vi "nanocal -- nuclear schottky fit V5.vi"() -> ()   [LabVIEW 2020] (continued)
\"mm3\" -> 0.000000000000   ,  \"T\" -> 1.000000000000   ,  \"B\" -> 0.000000000000   ,  \"θ\" -> 0.000000000000   ,  \"Reoff\" -> 0.000000000000   ,  \"Imoff\" -> 0.000000000000    |>   , \r\"IDS0220_210310_RAW_cal__ref_\" ->   <|    \"ζ\" -> 0.000000000000   ,  \"τ1\" -> 0.000000000000   ,  \"τS\" -> 0.000000000000   ,  \"τN\" -> 0.000000000000   ,  \"τC\" -> 0.000000000000   ,  \"κ0\" -> 0.000000000000   ,  \"mm1\" -> 0.000000000000   ,  \"mm2\" -> 0.000000000000   ,  \"mm3\" -> 0.000000000000   ,  \"T\" -> 0.677000000000   ,  \"B\" -> 0.000000000000   ,  \"θ\" -> 0.000000000000   ,  \"Reoff\" -> 0.000000000000   ,  \"Imoff\" -> 0.000000000000    |>   , \r\"IDS0220_210310_RAW_cal__sam_\" ->   <|    \"ζ\" -> 0.000000000000   ,  \"τ1\" -> 0.000000000000   ,  \"τS\" -> 0.000000000000   ,  \"τN\" -> 0.000000000000   ,  \"τC\" -> 0.000000000000   ,  \"κ0\" -> 0.000000000000   ,  \"mm1\" -> 0.000000000000   ,  \"mm2\" -> 0.000000000000   ,  \"mm3\" -> 0.000000000000   ,  \"T\" -> 0.677000000000   ,  \"B\" -> 0.000000000000   ,  \"θ\" -> 0.000000000000   ,  \"Reoff\" -> 0.000000000000   ,  \"Imoff\" -> 0.000000000000    |>   , \r\"IDS0224_210310_RAW_cal__ref_\" ->   <|    \"ζ\" -> 0.000000000000   ,  \"τ1\" -> 0.000000000000   ,  \"τS\" -> 0.000000000000   ,  \"τN\" -> 0.000000000000   ,  \"τC\" -> 0.000000000000   ,  \"κ0\" -> 0.000000000000   ,  \"mm1\" -> 0.000000000000   ,  \"mm2\" -> 0.000000000000   ,  \"mm3\" -> 0.000000000000   ,  \"T\" -> 0.000000000000   ,  \"B\" -> 0.000000000000   ,  \"θ\" -> 0.000000000000   ,  \"Reoff\" -> 0.000000000000   ,  \"Imoff\" -> 0.000000000000    |>   , \r\"IDS0224_210310_RAW_cal__sam_\" ->   <|    \"ζ\" -> 0.000000000000   ,  \"τ1\" -> 0.000000000000   ,  \"τS\" -> 0.000000000000   ,  \"τN\" -> 0.000000000000   ,  \"τC\" -> 0.000000000000   ,  \"κ0\" -> 0.000000000000   ,  \"mm1\" -> 0.000000000000   ,  \"mm2\" -> 0.000000000000   ,  \"mm3\" -> 0.000000000000   ,  \"T\" -> 0.000000000000   ,  \"B\" -> 0.000000000000   ,  \"θ\" -> 0.000000000000   ,  \"Reoff\" -> 0.000000000000   ,  \"Imoff\" -> 0.000000000000    |>   , \r\"IDS0293_210427_RAW_cal__ref_\" ->   <|    \"ζ\" -> 0.016384838586   ,  \"τ1\" -> 0.013784349529   ,  \"τS\" -> 0.011495286759   ,  \"τN\" -> 0.000117117954   ,  \"τC\" -> 0.004048153799   ,  \"κ0\" -> 0.000000013122   ,  \"mm1\" -> 0.000000000000   ,  \"mm2\" -> 0.000000000000   ,  \"mm3\" -> 0.000000000000   ,  \"T\" -> 1.900000000000   ,  \"B\" -> 12.000000000000   ,  \"θ\" -> 30.000000000000   ,  \"Reoff\" -> 0.000000000000   ,  \"Imoff\" -> 0.000000000000    |>   , \r\"IDS0293_210427_RAW_cal__sam_\" ->   <|    \"ζ\" -> 0.009772435939   ,  \"τ1\" -> 0.020827345370   ,  \"τS\" -> 0.013809334085   ,  \"τN\" -> 0.000168485133   ,  \"τC\" -> 0.005555066716   ,  \"κ0\" -> 0.000000013930   ,  \"mm1\" -> 0.000000000000   ,  \"mm2\" -> 0.000000000000   ,  \"mm3\" -> 0.000000000000   ,  \"T\" -> 1.900000000000   ,  \"B\" -> 12.000000000000   ,  \"θ\" -> 30.000000000000   ,  \"Reoff\" -> 0.000000000000   ,  \"Imoff\" -> 0.000000000000    |>   , \r\"IDS0294_210427_RAW_cal__ref_\" ->   <|    \"ζ\" -> 0.017975147456   ,  \"τ1\" -> 0.015573317032   ,  \"τS\" -> 0.016697357463   ,  \"τN\" -> 0.000401487663   ,  \"τC\" -> 0.004243374884   ,  \"κ0\" -> 0.000000007622   ,  \"mm1\" -> 0.000000000000   ,  \"mm2\" -> 0.000000000000   ,  \"mm3\" -> 0.000000000000   ,  \"T\" -> 1.130000000000   ,  \"B\" -> 12.000000000000   ,  \"θ\" -> 30.000000000000   ,  \"Reoff\" -> 0.000000000000   ,  \"Imoff\" -> 0.000000000000    |>   , \r\"IDS0294_210427_RAW_cal__sam_\" ->   <|    \"ζ\" -> 0.010912011148   ,  \"τ1\" -> 0.020760977312   ,  \"τS\" -> 0.021106239637   ,  \"τN\" -> 0.000452316988   ,  \"τC\" -> 0.005003723454   ,  \"κ0\" -> 0.000000008194   ,  \"mm1\" -> 0.000000000000   ,  \"mm2\" -> 0.000000000000   ,  \"mm3\" -> 0.000000000000   ,  \"T\" -> 1.130000000000   ,  \"B\" -> 12.000000000000   ,  \"θ\" -> 30.000000000000   ,  \"Reoff\" -> 0.000000000000   ,  \"Imoff\" -> 0.000000000000    |>   , \r\"IDS0295_210427_RAW_cal__ref_\" ->   <|    \"ζ\" -> 0.021360373560   ,  \"τ1\" -> 0.017226807214   ,  \"τS\" -> 0.021136224671   ,  \"τN\" -> 0.000857882935   ,  \"τC\" -> 0.004088468956   ,  \"κ0\" -> 0.000000005432   ,  \"mm1\" -> 0.000000000000   ,  \"mm2\" -> 0.000000000000   ,  \"mm3\" -> 0.000000000000   ,  \"T\" -> 0.830000000000   ,  \"B\" -> 12.000000000000   ,  \"θ\" -> 30.000000000000   ,  \"Reoff\" -> 0.000000000000   ,  \"Imoff\" -> 0.000000000000    |>   , \r\"IDS0295_210427_RAW_cal__sam_\" ->   <|    \"ζ\" -> 0.013460153434   ,  \"τ1\" -> 0.020684726260   ,  \"τS\" -> 0.027140346721   ,  \"τN\" -> 0.000960302406   ,  \"τC\" -> 0.004517434882   ,  \"κ0\" -> 0.000000005889   ,  \"mm1\" -> 0.000000000000   ,  \"mm2\" -> 0.000000000000   ,  \"mm3\" -> 0.000000000000   ,  \"T\" -> 0.830000000000   ,  \"B\" -> 12.000000000000   ,  \"θ\" -> 30.000000000000   ,  \"Reoff\" -> 0.000000000000   ,  \"Imoff\" -> 0.000000000000    |>   , \r\"IDS0296_210427_RAW_cal__ref_\" ->   <|    \"ζ\" -> 0.027756025784   ,  \"τ1\" -> 0.019742757718   ,  \"τS\" -> 0.026611973171   ,  \"τN\" -> 0.001398943183   ,  \"τC\" -> 0.003482574473   ,  \"κ0\" -> 0.000000003907   ,  \"mm1\" -> 0.000000000000   ,  \"mm2\" -> 0.000000000000   ,  \"mm3\" -> 0.000000000000   ,  \"T\" -> 0.620000000000   ,  \"B\" -> 12.000000000000   ,  \"θ\" -> 30.000000000000   ,  \"Reoff\" -> 0.000000000000   ,  \"Imoff\" -> 0.000000000000    |>   , \r\"IDS0296_210427_RAW_cal__sam_\" ->   <|    \"ζ\" -> 0.016892016292   ,  \"τ1\" -> 0.020344757415   ,  \"τS\" -> 0.033845756966   ,  \"τN\" -> 0.001946817417   ,  \"τC\" -> 0.004013762913   ,  \"κ0\" -> 0.000000004252   ,  \"mm1\" -> 0.000000000000   ,  \"mm2\" -> 0.000000000000   ,  \"mm3\" -> 0.000000000000   ,  \"T\" -> 0.620000000000   ,  \"B\" -> 12.000000000000   ,  \"θ\" -> 30.000000000000   ,  \"Reoff\" -> 0.000000000000   ,  \"Imoff\" -> 0.000000000000    |>   , \r\"IDS0297_210427_RAW_cal__ref_\" ->   <|    \"ζ\" -> 0.034775017342   ,  \"τ1\" -> 0.018923965005   ,  \"τS\" -> 0.030086686370   ,  \"τN\" -> 0.002286572055   ,  \"τC\" -> 0.002714831651   ,  \"κ0\" -> 0.000000003294   ,  \"mm1\" -> 0.000000000000   ,  \"mm2\" -> 0.000000000000   ,  \"mm3\" -> 0.000000000000   ,  \"T\" -> 0.530000000000   ,  \"B\" -> 12.000000000000   ,  \"θ\" -> 30.000000000000   ,  \"Reoff\" -> 0.000000000000   ,  \"Imoff\" -> 0.000000000000    |>   , \r\"IDS0297_210427_RAW_cal__sam_\" ->   <|    \"ζ\" -> 0.021116250068   ,  \"τ1\" -> 0.020669239851   ,  \"τS\" -> 0.037941648749   ,  \"τN\" -> 0.003221866945   ,  \"τC\" -> 0.003619427775   ,  \"κ0\" -> 0.000000003553   ,  \"mm1\" -> 0.000000000000   ,  \"mm2\" -> 0.000000000000   ,  \"mm3\" -> 0.000000000000   ,  \"T\" -> 0.530000000000   ,  \"B\" -> 12.000000000000   ,  \"θ\" -> 30.000000000000   ,  \"Reoff\" -> 0.000000000000   ,  \"Imoff\" -> 0.000000000000    |>   , \r\"IDS0298_210427_RAW_cal__ref_\" ->   <|    \"ζ\" -> 0.046396907778   ,  \"τ1\" -> 0.018912834926   ,  \"τS\" -> 0.034035556993   ,  \"τN\" -> 0.004466176128   ,  \"τC\" -> 0.002290347128   ,  \"κ0\" -> 0.000000002639   ,  \"mm1\" -> 0.000000000000   ,  \"mm2\" -> 0.000000000000   ,  \"mm3\" -> 0.000000000000   ,  \"T\" -> 0.430000000000   ,  \"B\" -> 12.000000000000   ,  \"θ\" -> 30.000000000000   ,  \"Reoff\" -> 0.000000000000   ,  \"Imoff\" -> 0.000000000000    |>   , \r\"IDS0298_210427_RAW_cal__sam_\" ->   <|    \"ζ\" -> 0.028468689077   ,  \"τ1\" -> 0.020220821810   ,  \"τS\" -> 0.043529484347   ,  \"τN\" -> 0.005653540941   ,  \"τC\" -> 0.003150537442   ,  \"κ0\" -> 0.000000002855   ,  \"mm1\" -> 0.000000000000   ,  \"mm2\" -> 0.000000000000   ,  \"mm3\" -> 0.000000000000   ,  \"T\" -> 0.430000000000   ,  \"B\" -> 12.000000000000   ,  \"θ\" -> 30.000000000000   ,  \"Reoff\" -> 0.000000000000   ,  \"Imoff\" -> 0.000000000000    |>   , \r\"IDS0299_210427_RAW_cal__ref_\" ->   <|    \"ζ\" -> 0.060257387765   ,  \"τ1\" -> 0.020933176342   ,  \"τS\" -> 0.038399909631   ,  \"τN\" -> 0.009014166994   ,  \"τC\" -> 0.001999715217   ,  \"κ0\" -> 0.000000002125   ,  \"mm1\" -> 0.000000000000   ,  \"mm2\" -> 0.000000000000   ,  \"mm3\" -> 0.000000000000   ,  \"T\" -> 0.360000000000   ,  \"B\" -> 12.000000000000   ,  \"θ\" -> 30.000000000000   ,  \"Reoff\" -> 0.000000000000   ,  \"Imoff\" -> 0.000000000000    |>   , \r\"IDS0299_210427_RAW_cal__sam_\" ->   <|    \"ζ\" -> 0.036420486357   ,  \"τ1\" -> 0.020986681106   ,  \"τS\" -> 0.049149577509   ,  \"τN\" -> 0.011109585503   ,  \"τC\" -> 0.002819780093   ,  \"κ0\" -> 0.000000002299   ,  \"mm1\" -> 0.000000000000   ,  \"mm2\" -> 0.000000000000   ,  \"mm3\" -> 0.000000000000   ,  \"T\" -> 0.360000000000   ,  \"B\" -> 12.000000000000   ,  \"θ\" -> 30.000000000000   ,  \"Reoff\" -> 0.000000000000   ,  \"Imoff\" -> 0.000000000000    |>   , \r\"IDS0300_210427_RAW_cal__ref_\" ->   <|    \"ζ\" -> 0.338385515343   ,  \"τ1\" -> 0.049005471612   ,  \"τS\" -> 0.154718584573   ,  \"τN\" -> 0.405362096342   ,  \"τC\" -> 0.001218418583   ,  \"κ0\" -> 0.000000000425   ,  \"mm1\" -> 0.000000000000   ,  \"mm2\" -> 0.000000000000   ,  \"mm3\" -> 0.000000000000   ,  \"T\" -> 0.140000000000   ,  \"B\" -> 12.000000000000   ,  \"θ\" -> 30.000000000000   ,  \"Reoff\" -> 0.000000000000   ,  \"Imoff\" -> 0.000000000000    |>   , \r\"IDS0300_210427_RAW_cal__sam_\" ->   <|    \"ζ\" -> 0.211545693132   ,  \"τ1\" -> 0.029106147473   ,  \"τS\" -> 0.094475691604   ,  \"τN\" -> 0.369151052631   ,  \"τC\" -> 0.001396700790   ,  \"κ0\" -> 0.000000000537   ,  \"mm1\" -> 0.000000000000   ,  \"mm2\" -> 0.000000000000   ,  \"mm3\" -> 0.000000000000   ,  \"T\" -> 0.140000000000   ,  \"B\" -> 12.000000000000   ,  \"θ\" -> 30.000000000000   ,  \"Reoff\" -> 0.000000000000   ,  \"Imoff\" -> 0.000000000000    |>   , \r\"IDS0301_210831_RAW_cal__ref_\" ->   <|    \"ζ\" -> 0.083856390991   ,  \"τ1\" -> 0.023882632275   ,  \"τS\" -> 0.042264558819   ,  \"τN\" -> 0.014926022610   ,  \"τC\" -> 0.001493479414   ,  \"κ0\" -> 0.000000001739   ,  \"mm1\" -> 0.000000000000   ,  \"mm2\" -> 0.000000000000   ,  \"mm3\" -> 0.000000000000   ,  \"T\" -> 0.300000000000   ,  \"B\" -> 12.000000000000   ,  \"θ\" -> 30.000000000000   ,  \"Reoff\" -> 0.000000000000   ,  \"Imoff\" -> 0.000000000000    |>   , \r\"IDS0301_210831_RAW_cal__sam_\" ->   <|    \"ζ\" -> 0.050663808076   ,  \"τ1\" -> 0.024940898568   ,  \"τS\" -> 0.056803871413   ,  \"τN\" -> 0.018856862265   ,  \"τC\" -> 0.002133501904   ,  \"κ0\" -> 0.000000001888   ,  \"mm1\" -> 0.000000000000   ,  \"mm2\" -> 0.000000000000   ,  \"mm3\" -> 0.000000000000   ,  \"T\" -> 0.300000000000   ,  \"B\" -> 12.000000000000   ,  \"θ\" -> 30.000000000000   ,  \"Reoff\" -> 0.000000000000   ,  \"Imoff\" -> 0.000000000000    |>   , \r\"IDS0302_210831_RAW_cal__ref_\" ->   <|    \"ζ\" -> 0.118191658932   ,  \"τ1\" -> 0.027786613255   ,  \"τS\" -> 0.049841575379   ,  \"τN\" -> 0.030683320319   ,  \"τC\" -> 0.001300754197   ,  \"κ0\" -> 0.000000001363   ,  \"mm1\" -> 0.000000000000   ,  \"mm2\" -> 0.000000000000   ,  \"mm3\" -> 0.000000000000   ,  \"T\" -> 0.250000000000   ,  \"B\" -> 12.000000000000   ,  \"θ\" -> 30.000000000000   ,  \"Reoff\" -> 0.000000000000   ,  \"Imoff\" -> 0.000000000000    |>   , \r\"IDS0302_210831_RAW_cal__sam_\" ->   <|    \"ζ\" -> 0.072634365939   ,  \"τ1\" -> 0.028637109000   ,  \"τS\" -> 0.065061142288   ,  \"τN\" -> 0.040304243071   ,  \"τC\" -> 0.001622979999   ,  \"κ0\" -> 0.000000001498   ,  \"mm1\" -> 0.000000000000   ,  \"mm2\" -> 0.000000000000   ,  \"mm3\" -> 0.000000000000   ,  \"T\" -> 0.250000000000   ,  \"B\" -> 12.000000000000   ,  \"θ\" -> 30.000000000000   ,  \"Reoff\" -> 0.000000000000   ,  \"Imoff\" -> 0.000000000000    |>   , \r\"IDS0303_210831_RAW_cal__ref_\" ->   <|    \"ζ\" -> 0.210185455037   ,  \"τ1\" -> 0.035884437188   ,  \"τS\" -> 0.076269858590   ,  \"τN\" -> 0.100000000000   ,  \"τC\" -> 0.001092094788   ,  \"κ0\" -> 0.000000001049   ,  \"mm1\" -> 0.000000000000   ,  \"mm2\" -> 0.000000000000   ,  \"mm3\" -> 0.000000000000   ,  \"T\" -> 0.200000000000   ,  \"B\" -> 12.000000000000   ,  \"θ\" -> 30.000000000000   ,  \"Reoff\" -> 0.000000000000   ,  \"Imoff\" -> 0.000000000000    |>   , \r\"IDS0303_210831_RAW_cal__sam_\" ->   <|    \"ζ\" -> 0.128615765969   ,  \"τ1\" -> 0.032665502211   ,  \"τS\" -> 0.082694869013   ,  \"τN\" -> 0.105788373632   ,  \"τC\" -> 0.001439686784   ,  \"κ0\" -> 0.000000001168   ,  \"mm1\" -> 0.000000000000   ,  \"mm2\" -> 0.000000000000   ,  \"mm3\" -> 0.000000000000   ,  \"T\" -> 0.200000000000   ,  \"B\" -> 12.000000000000   ,  \"θ\" -> 30.000000000000   ,  \"Reoff\" -> 0.000000000000   ,  \"Imoff\" -> 0.000000000000    |>   , \r\"IDS0304_210831_RAW_cal__ref_\" ->   <|    \"ζ\" -> 0.270205686716   ,  \"τ1\" -> 0.041964859676   ,  \"τS\" -> 0.093295997771   ,  \"τN\" -> 0.171907220186   ,  \"τC\" -> 0.001079705974   ,  \"κ0\" -> 0.000000000759   ,  \"mm1\" -> 0.000000000000   ,  \"mm2\" -> 0.000000000000   ,  \"mm3\" -> 0.000000000000   ,  \"T\" -> 0.170000000000   ,  \"B\" -> 12.000000000000   ,  \"θ\" -> 30.000000000000   ,  \"Reoff\" -> 0.000000000000   ,  \"Imoff\" -> 0.000000000000    |>   , \r\"IDS0304_210831_RAW_cal__sam_\" ->   <|    \"ζ\" -> 0.156472219566   ,  \"τ1\" -> 0.031017925061   ,  \"τS\" -> 0.080872234530   ,  \"τN\" -> 0.219381306397   ,  \"τC\" -> 0.001437792153   ,  \"κ0\" -> 0.000000000867   ,  \"mm1\" -> 0.000000000000   ,  \"mm2\" -> 0.000000000000   ,  \"mm3\" -> 0.000000000000   ,  \"T\" -> 0.170000000000   ,  \"B\" -> 12.000000000000   ,  \"θ\" -> 30.000000000000   ,  \"Reoff\" -> 0.000000000000   ,  \"Imoff\" -> 0.000000000000    |>   , \r\"IDS0305_210831_RAW_cal__ref_\" ->   <|    \"ζ\" -> 0.288872243536   ,  \"τ1\" -> 0.043051365220   ,  \"τS\" -> 0.113757726379   ,  \"τN\" -> 0.232280670982   ,  \"τC\" -> 0.001075362358   ,  \"κ0\" -> 0.000000000648   ,  \"mm1\" -> 0.000000000000   ,  \"mm2\" -> 0.000000000000   ,  \"mm3\" -> 0.000000000000   ,  \"T\" -> 0.160000000000   ,  \"B\" -> 12.000000000000   ,  \"θ\" -> 30.000000000000   ,  \"Reoff\" -> 0.000000000000   ,  \"Imoff\" -> 0.000000000000    |>   , \r\"IDS0305_210831_RAW_cal__sam_\" ->   <|    \"ζ\" -> 0.162585495535   ,  \"τ1\" -> 0.037883389730   ,  \"τS\" -> 0.086562863191   ,  \"τN\" -> 0.241872534356   ,  \"τC\" -> 0.001506143871   ,  \"κ0\" -> 0.000000000791   ,  \"mm1\" -> 0.000000000000   ,  \"mm2\" -> 0.000000000000   ,  \"mm3\" -> 0.000000000000   ,  \"T\" -> 0.160000000000   ,  \"B\" -> 12.000000000000   ,  \"θ\" -> 30.000000000000   ,  \"Reoff\" -> 0.000000000000   ,  \"Imoff\" -> 0.000000000000    |>   , \r\"IDS0306_210831_RAW_cal__ref_\" ->   <|    \"ζ\" -> 0.013593052641   ,  \"τ1\" -> 0.010989385662   ,  \"τS\" -> 0.007947176041   ,  \"τN\" -> 0.000037757079   ,  \"τC\" -> 0.003572854733   ,  \"κ0\" -> 0.000000023548   ,  \"mm1\" -> 0.000000000000   ,  \"mm2\" -> 0.000000000000   ,  \"mm3\" -> 0.000000000000   ,  \"T\" -> 3.100000000000   ,  \"B\" -> 12.000000000000   ,  \"θ\" -> 30.000000000000   ,  \"Reoff\" -> 0.000000000000   ,  \"Imoff\" -> 0.000000000000    |>   , \r\"IDS0306_210831_RAW_cal__sam_\" ->   <|    \"ζ\" -> 0.010111127240   ,  \"τ1\" -> 0.020788755574   ,  \"τS\" -> 0.009968978424   ,  \"τN\" -> 0.000077788811   ,  \"τC\" -> 0.004598584548   ,  \"κ0\" -> 0.000000024346   ,  \"mm1\" -> 0.000000000000   ,  \"mm2\" -> 0.000000000000   ,  \"mm3\" -> 0.000000000000   ,  \"T\" -> 3.100000000000   ,  \"B\" -> 12.000000000000   ,  \"θ\" -> 30.000000000000   ,  \"Reoff\" -> 0.000000000000   ,  \"Imoff\" -> 0.000000000000    |>   , \r\"IDS0310_210901_RAW_cal__ref_\" ->   <|    \"ζ\" -> 0.308289315544   ,  \"τ1\" -> 0.054346075620   ,  \"τS\" -> 0.066318547481   ,  \"τN\" -> 0.209207967486   ,  \"τC\" -> 0.001005266633   ,  \"κ0\" -> 0.000000000648   ,  \"mm1\" -> 0.000000000000   ,  \"mm2\" -> 0.000000000000   ,  \"mm3\" -> 0.000000000000   ,  \"T\" -> 0.157000000000   ,  \"B\" -> 12.000000000000   ,  \"θ\" -> 45.000000000000   ,  \"Reoff\" -> 0.000000000000   ,  \"Imoff\" -> 0.000000000000    |>   , \r\"IDS0310_210901_RAW_cal__sam_\" ->   <|    \"ζ\" -> 0.295520923520   ,  \"τ1\" -> 0.054772440405   ,  \"τS\" -> 0.071814005451   ,  \"τN\" -> 0.249593767169   ,  \"τC\" -> 0.001103632155   ,  \"κ0\" -> 0.000000000625   ,  \"mm1\" -> 0.000000000000   ,  \"mm2\" -> 0.000000000000   ,  \"mm3\" -> 0.000000000000   ,  \"T\" -> 0.157000000000   ,  \"B\" -> 12.000000000000   ,  \"θ\" -> 45.000000000000   ,  \"Reoff\" -> 0.000000000000   ,  \"Imoff\" -> 0.000000000000    |>   , \r\"IDS0311_210901_RAW_cal__ref_\" ->   <|    \"ζ\" -> 0.509291398058   ,  \"τ1\" -> 0.072489311123   ,  \"τS\" -> 0.090971238975   ,  \"τN\" -> 0.493344947632   ,  \"τC\" -> 0.000983845591   ,  \"κ0\" -> 0.000000000427   ,  \"mm1\" -> 0.000000000000   ,  \"mm2\" -> 0.000000000000   ,  \"mm3\" -> 0.000000000000   ,  \"T\" -> 0.120000000000   ,  \"B\" -> 12.000000000000   ,  \"θ\" -> 45.000000000000   ,  \"Reoff\" -> 0.000000000000   ,  \"Imoff\" -> 0.000000000000    |>   , \r\"IDS0311_210901_RAW_cal__sam_\" ->   <|    \"ζ\" -> 0.523545279740   ,  \"τ1\" -> 0.065613539167   ,  \"τS\" -> 0.100000000000   ,  \"τN\" -> 0.424083114177   ,  \"τC\" -> 0.000911255863   ,  \"κ0\" -> 0.000000000418   ,  \"mm1\" -> 0.000000000000   ,  \"mm2\" -> 0.000000000000   ,  \"mm3\" -> 0.000000000000   ,  \"T\" -> 0.120000000000   ,  \"B\" -> 12.000000000000   ,  \"θ\" -> 45.000000000000   ,  \"Reoff\" -> 0.000000000000   ,  \"Imoff\" -> 0.000000000000    |>   , \r\"IDS0312_210901_RAW_cal__ref_\" ->   <|    \"ζ\" -> 0.255987747016   ,  \"τ1\" -> 0.050915418179   ,  \"τS\" -> 0.056322890077   ,  \"τN\" -> 0.162539494258   ,  \"τC\" -> 0.001014478551   ,  \"κ0\" -> 0.000000000752   ,  \"mm1\" -> 0.000000000000   ,  \"mm2\" -> 0.000000000000   ,  \"mm3\" -> 0.000000000000   ,  \"T\" -> 0.170000000000   ,  \"B\" -> 12.000000000000   ,  \"θ\" -> 45.000000000000   ,  \"Reoff\" -> 0.000000000000   ,  \"Imoff\" -> 0.000000000000    |>   , \r\"IDS0312_210901_RAW_cal__sam_\" ->   <|    \"ζ\" -> 0.273742116471   ,  \"τ1\" -> 0.052262909995   ,  \"τS\" -> 0.060554036646   ,  \"τN\" -> 0.154269705680   ,  \"τC\" -> 0.001074144337   ,  \"κ0\" -> 0.000000000753   ,  \"mm1\" -> 0.000000000000   ,  \"mm2\" -> 0.000000000000   ,  \"mm3\" -> 0.000000000000   ,  \"T\" -> 0.170000000000   ,  \"B\" -> 12.000000000000   ,  \"θ\" -> 45.000000000000   ,  \"Reoff\" -> 0.000000000000   ,  \"Imoff\" -> 0.000000000000    |>   , \r\"IDS0313_210901_RAW_cal__ref_\" ->   <|    \"ζ\" -> 0.214174227031   ,  \"τ1\" -> 0.045371966885   ,  \"τS\" -> 0.046160741010   ,  \"τN\" -> 0.090352099204   ,  \"τC\" -> 0.001077653985   ,  \"κ0\" -> 0.000000001047   ,  \"mm1\" -> 0.000000000000   ,  \"mm2\" -> 0.000000000000   ,  \"mm3\" -> 0.000000000000   ,  \"T\" -> 0.200000000000   ,  \"B\" -> 12.000000000000   ,  \"θ\" -> 45.000000000000   ,  \"Reoff\" -> 0.000000000000   ,  \"Imoff\" -> 0.000000000000    |>   , \r\"IDS0313_210901_RAW_cal__sam_\" ->   <|    \"ζ\" -> 0.215688135788   ,  \"τ1\" -> 0.043710888546   ,  \"τS\" -> 0.044756474141   ,  \"τN\" -> 0.090222547904   ,  \"τC\" -> 0.001049781785   ,  \"κ0\" -> 0.000000001047   ,  \"mm1\" -> 0.000000000000   ,  \"mm2\" -> 0.000000000000   ,  \"mm3\" -> 0.000000000000   ,  \"T\" -> 0.200000000000   ,  \"B\" -> 12.000000000000   ,  \"θ\" -> 45.000000000000   ,  \"Reoff\" -> 0.000000000000   ,  \"Imoff\" -> 0.000000000000    |>   , \r\"IDS0314_210901_RAW_cal__ref_\" ->   <|    \"ζ\" -> 0.121938807235   ,  \"τ1\" -> 0.034207371807   ,  \"τS\" -> 0.036720955072   ,  \"τN\" -> 0.033836278502   ,  \"τC\" -> 0.001295467245   ,  \"κ0\" -> 0.000000001354   ,  \"mm1\" -> 0.000000000000   ,  \"mm2\" -> 0.000000000000   ,  \"mm3\" -> 0.000000000000   ,  \"T\" -> 0.255000000000   ,  \"B\" -> 12.000000000000   ,  \"θ\" -> 45.000000000000   ,  \"Reoff\" -> 0.000000000000   ,  \"Imoff\" -> 0.000000000000    |>   , \r\"IDS0314_210901_RAW_cal__sam_\" ->   <|    \"ζ\" -> 0.118583992968   ,  \"τ1\" -> 0.035232851003   ,  \"τS\" -> 0.037458022816   ,  \"τN\" -> 0.033724509363   ,  \"τC\" -> 0.001440922263   ,  \"κ0\" -> 0.000000001360   ,  \"mm1\" -> 0.000000000000   ,  \"mm2\" -> 0.000000000000   ,  \"mm3\" -> 0.000000000000   ,  \"T\" -> 0.255000000000   ,  \"B\" -> 12.000000000000   ,  \"θ\" -> 45.000000000000   ,  \"Reoff\" -> 0.000000000000   ,  \"Imoff\" -> 0.000000000000    |>   , \r\"IDS0315_210901_RAW_cal__ref_\" ->   <|    \"ζ\" -> 0.083994348522   ,  \"τ1\" -> 0.028454655874   ,  \"τS\" -> 0.032547522861   ,  \"τN\" -> 0.016695645368   ,  \"τC\" -> 0.001519868181   ,  \"κ0\" -> 0.000000001732   ,  \"mm1\" -> 0.000000000000   ,  \"mm2\" -> 0.000000000000   ,  \"mm3\" -> 0.000000000000   ,  \"T\" -> 0.300000000000   ,  \"B\" -> 12.000000000000   ,  \"θ\" -> 45.000000000000   ,  \"Reoff\" -> 0.000000000000   ,  \"Imoff\" -> 0.000000000000    |>   , \r\"IDS0315_210901_RAW_cal__sam_\" ->   <|    \"ζ\" -> 0.085152769414   ,  \"τ1\" -> 0.029001116263   ,  \"τS\" -> 0.032604663993   ,  \"τN\" -> 0.016878763935   ,  \"τC\" -> 0.001443524845   ,  \"κ0\" -> 0.000000001728   ,  \"mm1\" -> 0.000000000000   ,  \"mm2\" -> 0.000000000000   ,  \"mm3\" -> 0.000000000000   ,  \"T\" -> 0.300000000000   ,  \"B\" -> 12.000000000000   ,  \"θ\" -> 45.000000000000   ,  \"Reoff\" -> 0.000000000000   ,  \"Imoff\" -> 0.000000000000    |>   , \r\"IDS0316_210901_RAW_cal__ref_\" ->   <|    \"ζ\" -> 0.061161812807   ,  \"τ1\" -> 0.025679940958   ,  \"τS\" -> 0.030186846656   ,  \"τN\" -> 0.009745770789   ,  \"τC\" -> 0.001942458613   ,  \"κ0\" -> 0.000000002119   ,  \"mm1\" -> 0.000000000000   ,  \"mm2\" -> 0.000000000000   ,  \"mm3\" -> 0.000000000000   ,  \"T\" -> 0.360000000000   ,  \"B\" -> 12.000000000000   ,  \"θ\" -> 45.000000000000   ,  \"Reoff\" -> 0.000000000000   ,  \"Imoff\" -> 0.000000000000    |>   , \r\"IDS0316_210901_RAW_cal__sam_\" ->   <|    \"ζ\" -> 0.061011838044   ,  \"τ1\" -> 0.025440548989   ,  \"τS\" -> 0.030028053978   ,  \"τN\" -> 0.010140731955   ,  \"τC\" -> 0.001895079687   ,  \"κ0\" -> 0.000000002115   ,  \"mm1\" -> 0.000000000000   ,  \"mm2\" -> 0.000000000000   ,  \"mm3\" -> 0.000000000000   ,  \"T\" -> 0.360000000000   ,  \"B\" -> 12.000000000000   ,  \"θ\" -> 45.000000000000   ,  \"Reoff\" -> 0.000000000000   ,  \"Imoff\" -> 0.000000000000    |>   , \r\"IDS0317_210901_RAW_cal__ref_\" ->   <|    \"ζ\" -> 0.047188818117   ,  \"τ1\" -> 0.023281630947   ,  \"τS\" -> 0.027595934693   ,  \"τN\" -> 0.005357909158   ,  \"τC\" -> 0.002405018291   ,  \"κ0\" -> 0.000000002634   ,  \"mm1\" -> 0.000000000000   ,  \"mm2\" -> 0.000000000000   ,  \"mm3\" -> 0.000000000000   ,  \"T\" -> 0.430000000000   ,  \"B\" -> 12.000000000000   ,  \"θ\" -> 45.000000000000   ,  \"Reoff\" -> 0.000000000000   ,  \"Imoff\" -> 0.000000000000    |>   , \r\"IDS0317_210901_RAW_cal__sam_\" ->   <|    \"ζ\" -> 0.046686299518   ,  \"τ1\" -> 0.021011215626   ,  \"τS\" -> 0.027633142317   ,  \"τN\" -> 0.005348477555   ,  \"τC\" -> 0.002098477650   ,  \"κ0\" -> 0.000000002635   ,  \"mm1\" -> 0.000000000000   ,  \"mm2\" -> 0.000000000000   ,  \"mm3\" -> 0.000000000000   ,  \"T\" -> 0.430000000000   ,  \"B\" -> 12.000000000000   ,  \"θ\" -> 45.000000000000   ,  \"Reoff\" -> 0.000000000000   ,  \"Imoff\" -> 0.000000000000    |>   , \r\"IDS0318_210901_RAW_cal__ref_\" ->   <|    \"ζ\" -> 0.037288247068   ,  \"τ1\" -> 0.020701608824   ,  \"τS\" -> 0.025512873362   ,  \"τN\" -> 0.002622201076   ,  \"τC\" -> 0.002753838304   ,  \"κ0\" -> 0.000000003290   ,  \"mm1\" -> 0.000000000000   ,  \"mm2\" -> 0.000000000000   ,  \"mm3\" -> 0.000000000000   ,  \"T\" -> 0.530000000000   ,  \"B\" -> 12.000000000000   ,  \"θ\" -> 45.000000000000   ,  \"Reoff\" -> 0.000000000000   ,  \"Imoff\" -> 0.000000000000    |>   , \r\"IDS0318_210901_RAW_cal__sam_\" ->   <|    \"ζ\" -> 0.035204330012   ,  \"τ1\" -> 0.021011523093   ,  \"τS\" -> 0.025247316079   ,  \"τN\" -> 0.002718647875   ,  \"τC\" -> 0.003091727575   ,  \"κ0\" -> 0.000000003296   ,  \"mm1\" -> 0.000000000000   ,  \"mm2\" -> 0.000000000000   ,  \"mm3\" -> 0.000000000000   ,  \"T\" -> 0.530000000000   ,  \"B\" -> 12.000000000000   ,  \"θ\" -> 45.000000000000   ,  \"Reoff\" -> 0.000000000000   ,  \"Imoff\" -> 0.000000000000    |>   , \r\"IDS0319_210901_RAW_cal__ref_\" ->   <|    \"ζ\" -> 0.029057248634   ,  \"τ1\" -> 0.018506971535   ,  \"τS\" -> 0.023958337181   ,  \"τN\" -> 0.001609750825   ,  \"τC\" -> 0.003041346082   ,  \"κ0\" -> 0.000000003909   ,  \"mm1\" -> 0.000000000000   ,  \"mm2\" -> 0.000000000000   ,  \"mm3\" -> 0.000000000000   ,  \"T\" -> 0.620000000000   ,  \"B\" -> 12.000000000000   ,  \"θ\" -> 45.000000000000   ,  \"Reoff\" -> 0.000000000000   ,  \"Imoff\" -> 0.000000000000    |>   , \r\"IDS0319_210901_RAW_cal__sam_\" ->   <|    \"ζ\" -> 0.030862035723   ,  \"τ1\" -> 0.019328530751   ,  \"τS\" -> 0.023568572597   ,  \"τN\" -> 0.001701966614   ,  \"τC\" -> 0.003453790534   ,  \"κ0\" -> 0.000000003906   ,  \"mm1\" -> 0.000000000000   ,  \"mm2\" -> 0.000000000000   ,  \"mm3\" -> 0.000000000000   ,  \"T\" -> 0.620000000000   ,  \"B\" -> 12.000000000000   ,  \"θ\" -> 45.000000000000   ,  \"Reoff\" -> 0.000000000000   ,  \"Imoff\" -> 0.000000000000    |>   , \r\"IDS0320_210901_RAW_cal__ref_\" ->   <|    \"ζ\" -> 0.022379315068   ,  \"τ1\" -> 0.015662672554   ,  \"τS\" -> 0.020062485201   ,  \"τN\" -> 0.000750608517   ,  \"τC\" -> 0.004162319228   ,  \"κ0\" -> 0.000000005449   ,  \"mm1\" -> 0.000000000000   ,  \"mm2\" -> 0.000000000000   ,  \"mm3\" -> 0.000000000000   ,  \"T\" -> 0.830000000000   ,  \"B\" -> 12.000000000000   ,  \"θ\" -> 45.000000000000   ,  \"Reoff\" -> 0.000000000000   ,  \"Imoff\" -> 0.000000000000    |>   , \r\"IDS0320_210901_RAW_cal__sam_\" ->   <|    \"ζ\" -> 0.023591124045   ,  \"τ1\" -> 0.014910006225   ,  \"τS\" -> 0.019342950404   ,  \"τN\" -> 0.000752972387   ,  \"τC\" -> 0.004900413232   ,  \"κ0\" -> 0.000000005453   ,  \"mm1\" -> 0.000000000000   ,  \"mm2\" -> 0.000000000000   ,  \"mm3\" -> 0.000000000000   ,  \"T\" -> 0.830000000000   ,  \"B\" -> 12.000000000000   ,  \"θ\" -> 45.000000000000   ,  \"Reoff\" -> 0.000000000000   ,  \"Imoff\" -> 0.000000000000    |>   , \r\"IDS0321_210901_RAW_cal__ref_\" ->   <|    \"ζ\" -> 0.020614746765   ,  \"τ1\" -> 0.013682065369   ,  \"τS\" -> 0.016105139108   ,  \"τN\" -> 0.000397734649   ,  \"τC\" -> 0.005005824303   ,  \"κ0\" -> 0.000000007592   ,  \"mm1\" -> 0.000000000000   ,  \"mm2\" -> 0.000000000000   ,  \"mm3\" -> 0.000000000000   ,  \"T\" -> 1.130000000000   ,  \"B\" -> 12.000000000000   ,  \"θ\" -> 45.000000000000   ,  \"Reoff\" -> 0.000000000000   ,  \"Imoff\" -> 0.000000000000    |>   , \r\"IDS0321_210901_RAW_cal__sam_\" ->   <|    \"ζ\" -> 0.020215154826   ,  \"τ1\" -> 0.014105227254   ,  \"τS\" -> 0.015660924043   ,  \"τN\" -> 0.000525137036   ,  \"τC\" -> 0.005447728357   ,  \"κ0\" -> 0.000000007594   ,  \"mm1\" -> 0.000000000000   ,  \"mm2\" -> 0.000000000000   ,  \"mm3\" -> 0.000000000000   ,  \"T\" -> 1.130000000000   ,  \"B\" -> 12.000000000000   ,  \"θ\" -> 45.000000000000   ,  \"Reoff\" -> 0.000000000000   ,  \"Imoff\" -> 0.000000000000    |>   , \r\"IDS0322_210901_RAW_cal__ref_\" ->   <|    \"ζ\" -> 0.019557893298   ,  \"τ1\" -> 0.012446212333   ,  \"τS\" -> 0.011139553358   ,  \"τN\" -> 0.000114229396   ,  \"τC\" -> 0.005115315079   ,  \"κ0\" -> 0.000000013115   ,  \"mm1\" -> 0.000000000000   ,  \"mm2\" -> 0.000000000000   ,  \"mm3\" -> 0.000000000000   ,  \"T\" -> 1.900000000000   ,  \"B\" -> 12.000000000000   ,  \"θ\" -> 45.000000000000   ,  \"Reoff\" -> 0.000000000000   ,  \"Imoff\" -> 0.000000000000    |>   , \r\"IDS0322_210901_RAW_cal__sam_\" ->   <|    \"ζ\" -> 0.018090572724   ,  \"τ1\" -> 0.013314780956   ,  \"τS\" -> 0.010820835010   ,  \"τN\" -> 0.000265552167   ,  \"τC\" -> 0.005393540417   ,  \"κ0\" -> 0.000000013100   ,  \"mm1\" -> 0.000000000000   ,  \"mm2\" -> 0.000000000000   ,  \"mm3\" -> 0.000000000000   ,  \"T\" -> 1.900000000000   ,  \"B\" -> 12.000000000000   ,  \"θ\" -> 45.000000000000   ,  \"Reoff\" -> 0.000000000000   ,  \"Imoff\" -> 0.000000000000    |>   , \r\"IDS0323_210901_RAW_cal__ref_\" ->   <|    \"ζ\" -> 0.018290634783   ,  \"τ1\" -> 0.011707989393   ,  \"τS\" -> 0.007391181448   ,  \"τN\" -> 0.000042685582   ,  \"τC\" -> 0.004638632451   ,  \"κ0\" -> 0.000000023525   ,  \"mm1\" -> 0.000000000000   ,  \"mm2\" -> 0.000000000000   ,  \"mm3\" -> 0.000000000000   ,  \"T\" -> 3.100000000000   ,  \"B\" -> 12.000000000000   ,  \"θ\" -> 45.000000000000   ,  \"Reoff\" -> 0.000000000000   ,  \"Imoff\" -> 0.000000000000    |>   , \r\"IDS0323_210901_RAW_cal__sam_\" ->   <|    \"ζ\" -> 0.019438138135   ,  \"τ1\" -> 0.013521019406   ,  \"τS\" -> 0.007253169401   ,  \"τN\" -> 0.000154824830   ,  \"τC\" -> 0.004746579385   ,  \"κ0\" -> 0.000000023466   ,  \"mm1\" -> 0.000000000000   ,  \"mm2\" -> 0.000000000000   ,  \"mm3\" -> 0.000000000000   ,  \"T\" -> 3.100000000000   ,  \"B\" -> 12.000000000000   ,  \"θ\" -> 45.000000000000   ,  \"Reoff\" -> 0.000000000000   ,  \"Imoff\" -> 0.000000000000    |>   , \r\"IDS0324_210901_RAW_cal__ref_\" ->   <|    \"ζ\" -> 0.016342153608   ,  \"τ1\" -> 0.012470308436   ,  \"τS\" -> 0.004793459347   ,  \"τN\" -> 0.000012881713   ,  \"τC\" -> 0.003213848745   ,  \"κ0\" -> 0.000000058321   ,  \"mm1\" -> 0.000000000000   ,  \"mm2\" -> 0.000000000000   ,  \"mm3\" -> 0.000000000000   ,  \"T\" -> 5.700000000000   ,  \"B\" -> 12.000000000000   ,  \"θ\" -> 45.000000000000   ,  \"Reoff\" -> 0.000000000000   ,  \"Imoff\" -> 0.000000000000    |>   , \r\"IDS0324_210901_RAW_cal__sam_\" ->   <|    \"ζ\" -> 0.018573189054   ,  \"τ1\" -> 0.013304612245   ,  \"τS\" -> 0.003723860844   ,  \"τN\" -> 0.000084829442   ,  \"τC\" -> 0.004309703632   ,  \"κ0\" -> 0.000000058362   ,  \"mm1\" -> 0.000000000000   ,  \"mm2\" -> 0.000000000000   ,  \"mm3\" -> 0.000000000000   ,  \"T\" -> 5.700000000000   ,  \"B\" -> 12.000000000000   ,  \"θ\" -> 45.000000000000   ,  \"Reoff\" -> 0.000000000000   ,  \"Imoff\" -> 0.000000000000    |>   , \r\"IDS0330_210901_RAW_cal__ref_\" ->   <|    \"ζ\" -> 0.000000000000   ,  \"τ1\" -> 0.000000000000   ,  \"τS\" -> 0.000000000000   ,  \"τN\" -> 0.000000000000   ,  \"τC\" -> 0.000000000000   ,  \"κ0\" -> 0.000000000000   ,  \"mm1\" -> 0.000000000000   ,  \"mm2\" -> 0.000000000000   ,  \"mm3\" -> 0.000000000000   ,  \"T\" -> 0.197000000000   ,  \"B\" -> 1.000000000000   ,  \"θ\" -> 90.000000000000   ,  \"Reoff\" -> 0.000000000000   ,  \"Imoff\" -> 0.000000000000    |>   , \r\"IDS0330_210901_RAW_cal__sam_\" ->   <|    \"ζ\" -> 0.000000000000   ,  \"τ1\" -> 0.000000000000   ,  \"τS\" -> 0.000000000000   ,  \"τN\" -> 0.000000000000   ,  \"τC\" -> 0.000000000000   ,  \"κ0\" -> 0.000000000000   ,  \"mm1\" -> 0.000000000000   ,  \"mm2\" -> 0.000000000000   ,  \"mm3\" -> 0.000000000000   ,  \"T\" -> 0.197000000000   ,  \"B\" -> 1.000000000000   ,  \"θ\" -> 90.000000000000   ,  \"Reoff\" -> 0.000000000000   ,  \"Imoff\" -> 0.000000000000    |>   , \r\"IDS0331_210901_RAW_cal__ref_\" ->   <|    \"ζ\" -> 0.000000000000   ,  \"τ1\" -> 0.000000000000   ,  \"τS\" -> 0.000000000000   ,  \"τN\" -> 0.000000000000   ,  \"τC\" -> 0.000000000000   ,  \"κ0\" -> 0.000000000000   ,  \"mm1\" -> 0.000000000000   ,  \"mm2\" -> 0.000000000000   ,  \"mm3\" -> 0.000000000000   ,  \"T\" -> 0.197000000000   ,  \"B\" -> 2.000000000000   ,  \"θ\" -> 90.000000000000   ,  \"Reoff\" -> 0.000000000000   ,  \"Imoff\" -> 0.000000000000    |>   , \r\"IDS0331_210901_RAW_cal__sam_\" ->   <|    \"ζ\" -> 0.000000000000   ,  \"τ1\" -> 0.000000000000   ,  \"τS\" -> 0.000000000000   ,  \"τN\" -> 0.000000000000   ,  \"τC\" -> 0.000000000000   ,  \"κ0\" -> 0.000000000000   ,  \"mm1\" -> 0.000000000000   ,  \"mm2\" -> 0.000000000000   ,  \"mm3\" -> 0.000000000000   ,  \"T\" -> 0.197000000000   ,  \"B\" -> 2.000000000000   ,  \"θ\" -> 90.000000000000   ,  \"Reoff\" -> 0.000000000000   ,  \"Imoff\" -> 0.000000000000    |>   , \r\"IDS0335_210904_RAW_cal__ref_\" ->   <|    \"ζ\" -> 0.208053746206   ,  \"τ1\" -> 0.038411915919   ,  \"τS\" -> 0.085156832322   ,  \"τN\" -> 0.009965050261   ,  \"τC\" -> 0.001092766705   ,  \"κ0\" -> 0.000000001027   ,  \"mm1\" -> 0.000000000000   ,  \"mm2\" -> 0.000000000000   ,  \"mm3\" -> 0.000000000000   ,  \"T\" -> 0.197000000000   ,  \"B\" -> 5.000000000000   ,  \"θ\" -> 90.000000000000   ,  \"Reoff\" -> -30047029.702970296200   ,  \"Imoff\" -> 0.000000000000    |>   , \r\"IDS0335_210904_RAW_cal__sam_\" ->   <|    \"ζ\" -> 0.126082356467   ,  \"τ1\" -> 0.023836839175   ,  \"τS\" -> 0.108299123409   ,  \"τN\" -> 0.016157535301   ,  \"τC\" -> 0.001495872883   ,  \"κ0\" -> 0.000000001129   ,  \"mm1\" -> 0.000000000000   ,  \"mm2\" -> 0.000000000000   ,  \"mm3\" -> 0.000000000000   ,  \"T\" -> 0.197000000000   ,  \"B\" -> 5.000000000000   ,  \"θ\" -> 90.000000000000   ,  \"Reoff\" -> 0.000000000000   ,  \"Imoff\" -> 0.000000000000    |>   , \r\"IDS0336_210904_RAW_cal__ref_\" ->   <|    \"ζ\" -> 0.382189262063   ,  \"τ1\" -> 0.053460340134   ,  \"τS\" -> 0.186079633695   ,  \"τN\" -> 0.081484000727   ,  \"τC\" -> 0.001241323487   ,  \"κ0\" -> 0.000000000381   ,  \"mm1\" -> 0.000000000000   ,  \"mm2\" -> 0.000000000000   ,  \"mm3\" -> 0.000000000000   ,  \"T\" -> 0.122000000000   ,  \"B\" -> 5.000000000000   ,  \"θ\" -> 90.000000000000   ,  \"Reoff\" -> -105086633.663366333000   ,  \"Imoff\" -> 0.000000000000    |>   , \r\"IDS0336_210904_RAW_cal__sam_\" ->   <|    \"ζ\" -> 0.192483765517   ,  \"τ1\" -> 0.026761797789   ,  \"τS\" -> 0.278068103221   ,  \"τN\" -> 0.092231648139   ,  \"τC\" -> 0.001612694918   ,  \"κ0\" -> 0.000000000500   ,  \"mm1\" -> 0.000000000000   ,  \"mm2\" -> 0.000000000000   ,  \"mm3\" -> 0.000000000000   ,  \"T\" -> 0.122000000000   ,  \"B\" -> 5.000000000000   ,  \"θ\" -> 90.000000000000   ,  \"Reoff\" -> 0.000000000000   ,  \"Imoff\" -> 0.000000000000    |>   , \r\"IDS0337_210904_RAW_cal__ref_\" ->   <|    \"ζ\" -> 0.286155958451   ,  \"τ1\" -> 0.040795360167   ,  \"τS\" -> 0.124676030229   ,  \"τN\" -> 0.028515892527   ,  \"τC\" -> 0.001166840208   ,  \"κ0\" -> 0.000000000640   ,  \"mm1\" -> 0.000000000000   ,  \"mm2\" -> 0.000000000000   ,  \"mm3\" -> 0.000000000000   ,  \"T\" -> 0.157000000000   ,  \"B\" -> 5.000000000000   ,  \"θ\" -> 90.000000000000   ,  \"Reoff\" -> -56123762.376237616000   ,  \"Imoff\" -> 0.000000000000    |>   , \r\"IDS0337_210904_RAW_cal__sam_\" ->   <|    \"ζ\" -> 0.176757536135   ,  \"τ1\" -> 0.025030443527   ,  \"τS\" -> 0.157985418261   ,  \"τN\" -> 0.029253173903   ,  \"τC\" -> 0.001444377194   ,  \"κ0\" -> 0.000000000743   ,  \"mm1\" -> 0.000000000000   ,  \"mm2\" -> 0.000000000000   ,  \"mm3\" -> 0.000000000000   ,  \"T\" -> 0.157000000000   ,  \"B\" -> 5.000000000000   ,  \"θ\" -> 90.000000000000   ,  \"Reoff\" -> 0.000000000000   ,  \"Imoff\" -> 0.000000000000    |>   , \r\"IDS0338_210904_RAW_cal__ref_\" ->   <|    \"ζ\" -> 0.269546283128   ,  \"τ1\" -> 0.045502488609   ,  \"τS\" -> 0.108672194681   ,  \"τN\" -> 0.019017589637   ,  \"τC\" -> 0.001052941026   ,  \"κ0\" -> 0.000000000729   ,  \"mm1\" -> 0.000000000000   ,  \"mm2\" -> 0.000000000000   ,  \"mm3\" -> 0.000000000000   ,  \"T\" -> 0.170000000000   ,  \"B\" -> 5.000000000000   ,  \"θ\" -> 90.000000000000   ,  \"Reoff\" -> -56123762.376237616000   ,  \"Imoff\" -> 0.000000000000    |>   , \r\"IDS0338_210904_RAW_cal__sam_\" ->   <|    \"ζ\" -> 0.157490327814   ,  \"τ1\" -> 0.025072576319   ,  \"τS\" -> 0.138913916780   ,  \"τN\" -> 0.024096402149   ,  \"τC\" -> 0.001407824448   ,  \"κ0\" -> 0.000000000841   ,  \"mm1\" -> 0.000000000000   ,  \"mm2\" -> 0.000000000000   ,  \"mm3\" -> 0.000000000000   ,  \"T\" -> 0.170000000000   ,  \"B\" -> 5.000000000000   ,  \"θ\" -> 90.000000000000   ,  \"Reoff\" -> 0.000000000000   ,  \"Imoff\" -> 0.000000000000    |>   , \r\"IDS0339_210904_RAW_cal__ref_\" ->   <|    \"ζ\" -> 0.118077525137   ,  \"τ1\" -> 0.030857488721   ,  \"τS\" -> 0.060111159866   ,  \"τN\" -> 0.005614896894   ,  \"τC\" -> 0.001326778758   ,  \"κ0\" -> 0.000000001340   ,  \"mm1\" -> 0.000000000000   ,  \"mm2\" -> 0.000000000000   ,  \"mm3\" -> 0.000000000000   ,  \"T\" -> 0.255000000000   ,  \"B\" -> 5.000000000000   ,  \"θ\" -> 90.000000000000   ,  \"Reoff\" -> -13995049.504950495400   ,  \"Imoff\" -> 0.000000000000    |>   , \r\"IDS0339_210904_RAW_cal__sam_\" ->   <|    \"ζ\" -> 0.071547151941   ,  \"τ1\" -> 0.023411099214   ,  \"τS\" -> 0.077624659702   ,  \"τN\" -> 0.006792929714   ,  \"τC\" -> 0.001758131380   ,  \"κ0\" -> 0.000000001477   ,  \"mm1\" -> 0.000000000000   ,  \"mm2\" -> 0.000000000000   ,  \"mm3\" -> 0.000000000000   ,  \"T\" -> 0.255000000000   ,  \"B\" -> 5.000000000000   ,  \"θ\" -> 90.000000000000   ,  \"Reoff\" -> 0.000000000000   ,  \"Imoff\" -> 0.000000000000    |>   , \r\"IDS0340_210904_RAW_cal__ref_\" ->   <|    \"ζ\" -> 0.081700724360   ,  \"τ1\" -> 0.030900177229   ,  \"τS\" -> 0.049782214826   ,  \"τN\" -> 0.003013726898   ,  \"τC\" -> 0.001578655445   ,  \"κ0\" -> 0.000000001717   ,  \"mm1\" -> 0.000000000000   ,  \"mm2\" -> 0.000000000000   ,  \"mm3\" -> 0.000000000000   ,  \"T\" -> 0.308000000000   ,  \"B\" -> 5.000000000000   ,  \"θ\" -> 90.000000000000   ,  \"Reoff\" -> -7351485.148514851930   ,  \"Imoff\" -> 0.000000000000    |>   , \r\"IDS0340_210904_RAW_cal__sam_\" ->   <|    \"ζ\" -> 0.049129914970   ,  \"τ1\" -> 0.024898573189   ,  \"τS\" -> 0.064441011576   ,  \"τN\" -> 0.003850324949   ,  \"τC\" -> 0.002205260995   ,  \"κ0\" -> 0.000000001876   ,  \"mm1\" -> 0.000000000000   ,  \"mm2\" -> 0.000000000000   ,  \"mm3\" -> 0.000000000000   ,  \"T\" -> 0.308000000000   ,  \"B\" -> 5.000000000000   ,  \"θ\" -> 90.000000000000   ,  \"Reoff\" -> 0.000000000000   ,  \"Imoff\" -> 0.000000000000    |>   , \r\"IDS0341_210904_RAW_cal__ref_\" ->   <|    \"ζ\" -> 0.060181637857   ,  \"τ1\" -> 0.031657037942   ,  \"τS\" -> 0.042859576552   ,  \"τN\" -> 0.001817067710   ,  \"τC\" -> 0.001921890953   ,  \"κ0\" -> 0.000000002089   ,  \"mm1\" -> 0.000000000000   ,  \"mm2\" -> 0.000000000000   ,  \"mm3\" -> 0.000000000000   ,  \"T\" -> 0.360000000000   ,  \"B\" -> 5.000000000000   ,  \"θ\" -> 90.000000000000   ,  \"Reoff\" -> -3878712.871287129820   ,  \"Imoff\" -> 0.000000000000    |>   , \r\"IDS0341_210904_RAW_cal__sam_\" ->   <|    \"ζ\" -> 0.036232012390   ,  \"τ1\" -> 0.027781521532   ,  \"τS\" -> 0.055391702939   ,  \"τN\" -> 0.001971026378   ,  \"τC\" -> 0.002721128929   ,  \"κ0\" -> 0.000000002279   ,  \"mm1\" -> 0.000000000000   ,  \"mm2\" -> 0.000000000000   ,  \"mm3\" -> 0.000000000000   ,  \"T\" -> 0.360000000000   ,  \"B\" -> 5.000000000000   ,  \"θ\" -> 90.000000000000   ,  \"Reoff\" -> 0.000000000000   ,  \"Imoff\" -> 0.000000000000    |>   , \r\"IDS0342_210904_RAW_cal__ref_\" ->   <|    \"ζ\" -> 0.044382820544   ,  \"τ1\" -> 0.023962063047   ,  \"τS\" -> 0.036003766802   ,  \"τN\" -> 0.001081378527   ,  \"τC\" -> 0.002322219341   ,  \"κ0\" -> 0.000000002628   ,  \"mm1\" -> 0.000000000000   ,  \"mm2\" -> 0.000000000000   ,  \"mm3\" -> 0.000000000000   ,  \"T\" -> 0.438000000000   ,  \"B\" -> 5.000000000000   ,  \"θ\" -> 90.000000000000   ,  \"Reoff\" -> -2393564.356435643510   ,  \"Imoff\" -> 0.000000000000    |>   , \r\"IDS0342_210904_RAW_cal__sam_\" ->   <|    \"ζ\" -> 0.029055572135   ,  \"τ1\" -> 0.027337777983   ,  \"τS\" -> 0.046740216600   ,  \"τN\" -> 0.000913387218   ,  \"τC\" -> 0.003013145103   ,  \"κ0\" -> 0.000000002847   ,  \"mm1\" -> 0.000000000000   ,  \"mm2\" -> 0.000000000000   ,  \"mm3\" -> 0.000000000000   ,  \"T\" -> 0.438000000000   ,  \"B\" -> 5.000000000000   ,  \"θ\" -> 90.000000000000   ,  \"Reoff\" -> 0.000000000000   ,  \"Imoff\" -> 0.000000000000    |>   , \r\"IDS0343_210904_RAW_cal__ref_\" ->   <|    \"ζ\" -> 0.035716753589   ,  \"τ1\" -> 0.022977795767   ,  \"τS\" -> 0.030561871473   ,  \"τN\" -> 0.000475699989   ,  \"τC\" -> 0.002838061607   ,  \"κ0\" -> 0.000000003273   ,  \"mm1\" -> 0.000000000000   ,  \"mm2\" -> 0.000000000000   ,  \"mm3\" -> 0.000000000000   ,  \"T\" -> 0.530000000000   ,  \"B\" -> 5.000000000000   ,  \"θ\" -> 90.000000000000   ,  \"Reoff\" -> -1735148.514851485150   ,  \"Imoff\" -> 0.000000000000    |>   , \r\"IDS0343_210904_RAW_cal__sam_\" ->   <|    \"ζ\" -> 0.023052185319   ,  \"τ1\"
